vi "DE_Update State.vi"(8 "error in (no error)":errorcluster, 9 "State In":T1, 11 "Candidate State":T1) -> (0 "error out":errorcluster, 1 "State Out":T1)   [LabVIEW 2020, in "NI_AAL_GlobalOptimization.lvlib"]
uses:
  <vilib>/gmath/NI_AAL_GlobalOptimization.lvlib
  <vilib>/gmath/GlobalOptimization.llb/DE_State.ctl
  <vilib>/gmath/GlobalOptimization.llb/DE_Population.ctl
  <vilib>/gmath/GlobalOptimization.llb/DE_Population Comparison.ctl
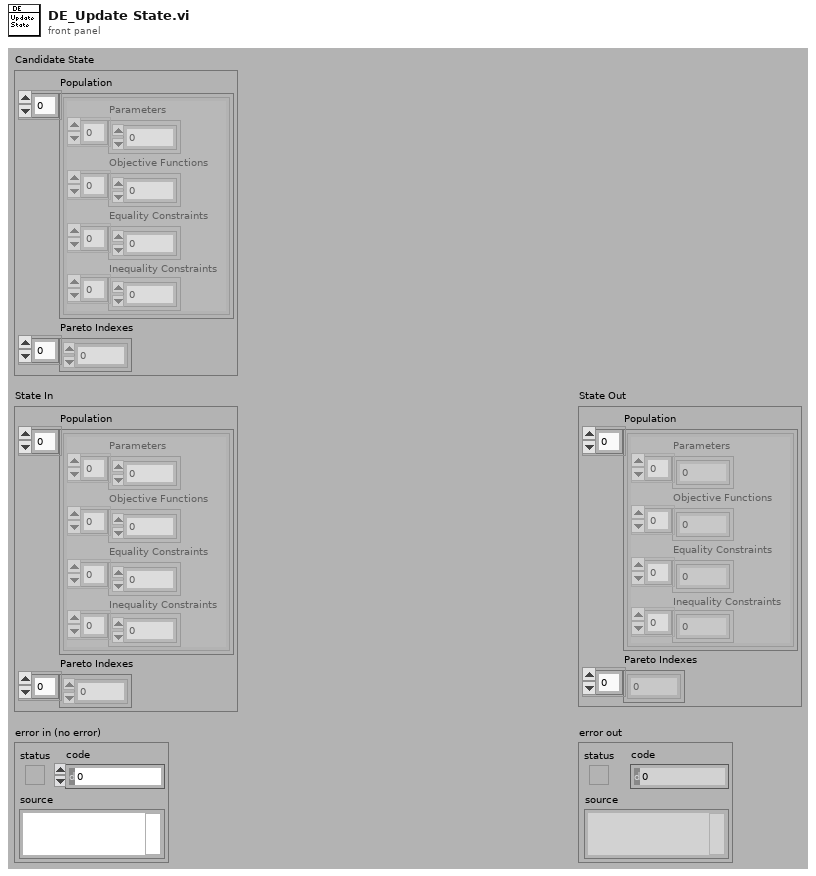
[diagram p1: front panel]
types:
  T1 = typedef "NI_AAL_GlobalOptimization.lvlib/DE_State.ctl" = cluster{"Population":T2[], "Pareto Indexes":i32[]}
  T2 = typedef "NI_AAL_GlobalOptimization.lvlib/DE_Population.ctl" = cluster{"Parameters":dbl[], "Objective Functions":dbl[], "Equality Constraints":dbl[], "Inequality Constraints":dbl[]}
  T3 = typedef "NI_AAL_GlobalOptimization.lvlib/DE_Population Comparison.ctl" = u16
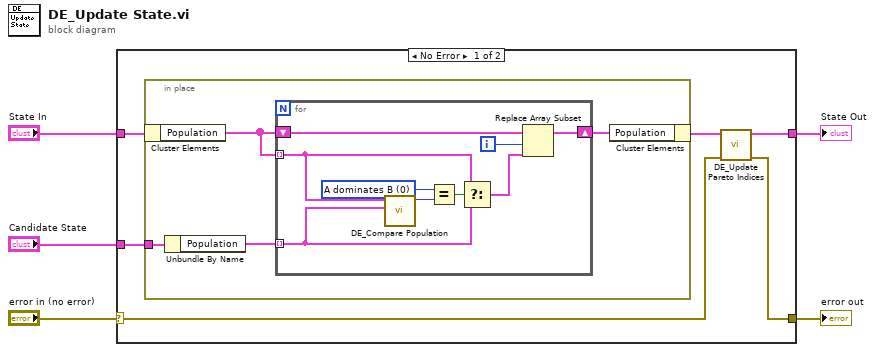
[diagram p0: block diagram]
diagram:
  n1 = case shown="No Error" "error in (no error)" {
    selector: "error in (no error)" -> [w8 w25]
    tunnel: "State In" -> [w7 w26]
    tunnel: "Candidate State" -> [w11 _]
    tunnel: [w10 w26] -> w3
    tunnel: [w9 w25] -> w1
    frame No Error {
      n2 = in-place {
        in-place-border: w11 -> [w15]
        n3 = in-place-cluster #1(w7) -> ("Population"=w13:T2[])
        n4 = Unbundle By Name(w15) -> ("Population"=w14:T2[])
        n5 = for {
          tunnel: w13 -> [w21] mode=indexing
          tunnel: w14 -> [w20] mode=indexing
          shift-right: [w17] -> w12
          shift-left: w13 -> [w19]
          i -> [w16]
          w23 = T3 0 items=["A dominates B", "B dominates A", "Neither dominates", "A = B"] ("x")
          n6 = call <vilib>:"DE_Compare Population.vi"("Population B"=w20, "Population A"=w21) -> ("population comparison"=w24:T3)  [unwired: 8 in, 1 out]
          n7 = Equal?(x=w23, y=w24) -> (x = y?=w22:bool)
          n8 = Select(t=w21, s=w22, f=w20) -> (s? t:f=w18:T2)
          n9 = Replace Array Subset(array=w19, new element=w18, index=w16) -> (w17:T2[])
        }
        n10 = in-place-cluster #1("Population"=w12) -> (w6:T1)
      }
      n11 = call <vilib>:"DE_Update Pareto Indices.vi"("error in (no error)"=w8, "State In"=w6) -> ("error out"=w9:errorcluster, "State Out"=w10:T1)  [unwired: 7 in, 1 out]
    }
    frame Error {
    }
  }
  "error out" <- w1
  "State Out" <- w3
